vi "Calculator_Main.vi"() -> ()   [LabVIEW 2017]
uses:
  Controls/Calculator_States.ctl
  Controls/Master_Cluster.ctl
panel:
  out "Result":dbl
  out "Data Entry":string
  in  "Button 17":bool
  in  "DIV":bool
  in  "Button 21":bool
  in  "Button 20":bool
  in  "Button 19":bool
  in  "Button 18":bool
  in  "MUL":bool
  in  "SUB":bool
  in  "ADD":bool
  in  "Equals":bool
  in  "NUM 9":bool
  in  "NUM 8":bool
  in  "NUM 7":bool
  in  "NUM 6":bool
  in  "NUM 5":bool
  in  "NUM 4":bool
  in  "NUM 3":bool
  in  "NUM 2":bool
  in  "NUM 1":bool
  in  "Period":bool
  in  "NUM 0":bool
  in  "Button 1":bool
  in  "Exit":bool
  out "error out":errorcluster
  in  "error in (no error)":errorcluster
  # "CALCULATOR"
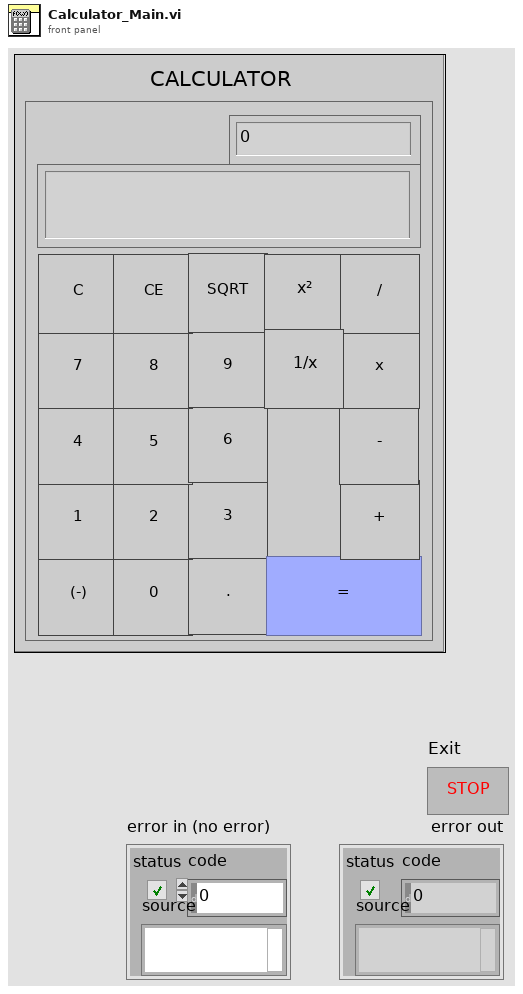
[diagram p1: front panel]
types:
  T1 = typedef "Calculator_States.ctl" = enum16{"Poll", "Initialise", "Update Data Entry", "Update Result", "Update Indicators", "Error", "Exit"}
  T2 = typedef "Master_Cluster.ctl" = cluster{"Data Entry Array":string[], "Data Entry Display":string, "Before Operator":dbl, "After Operator":dbl, "Result":dbl, "Operator":string}
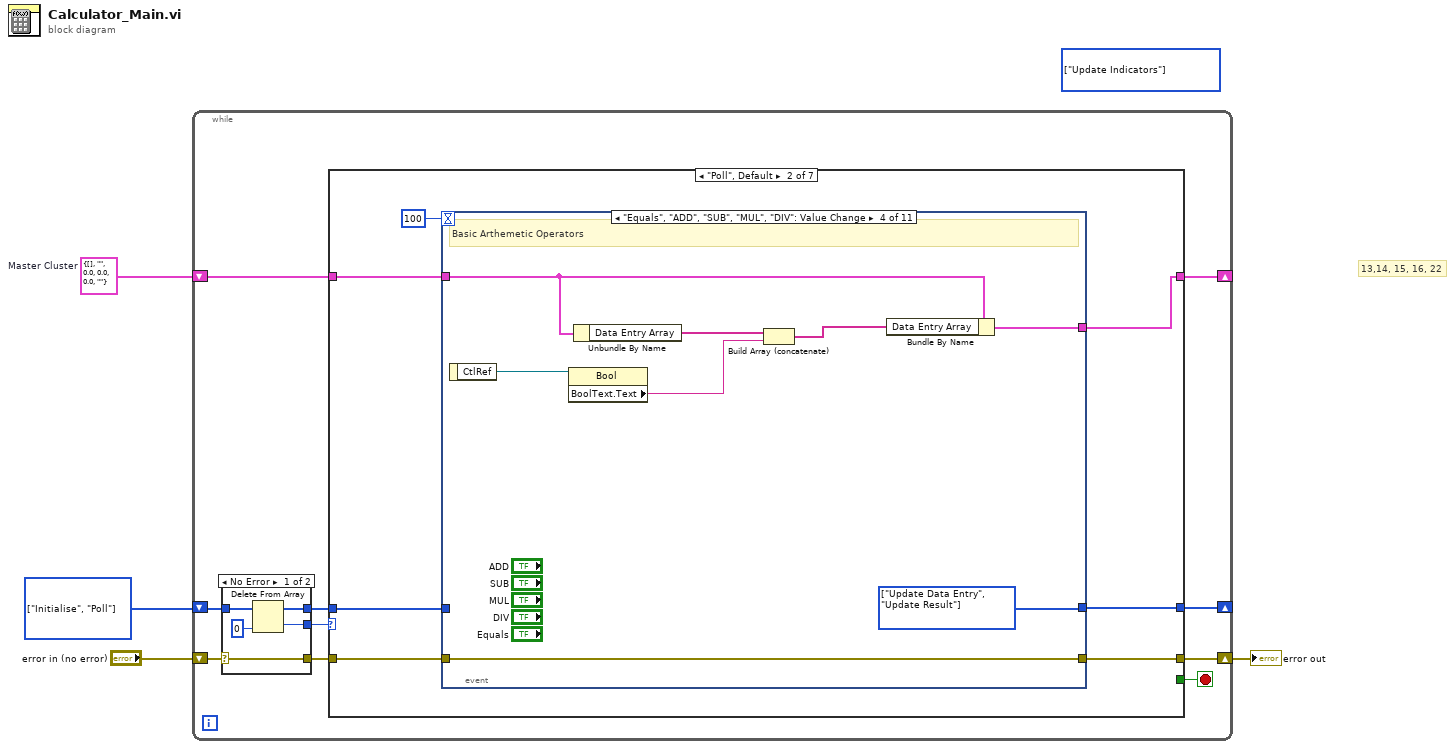
[diagram p0: block diagram]
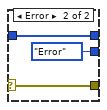
[diagram p2: hidden frame]
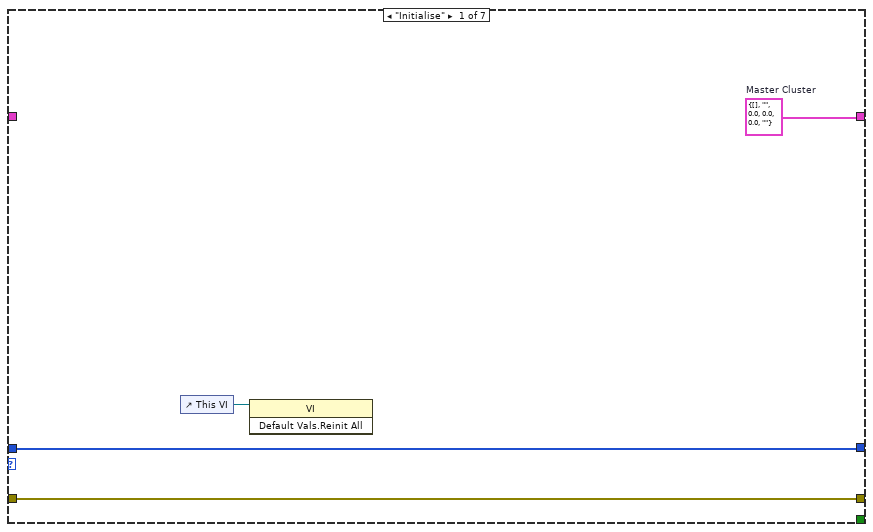
[diagram p3: hidden frame]
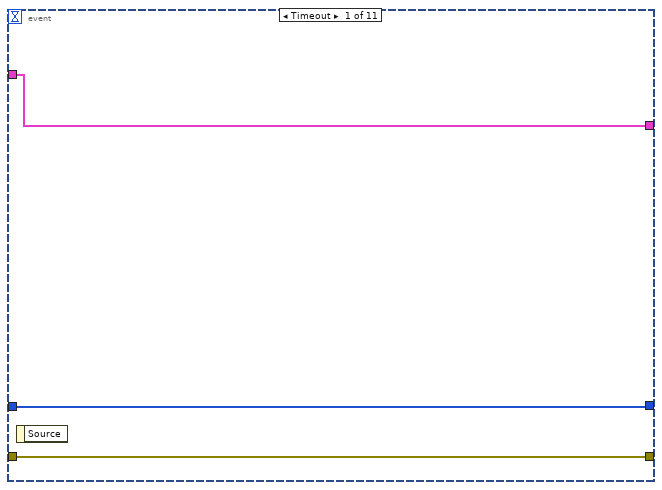
[diagram p4: hidden frame]
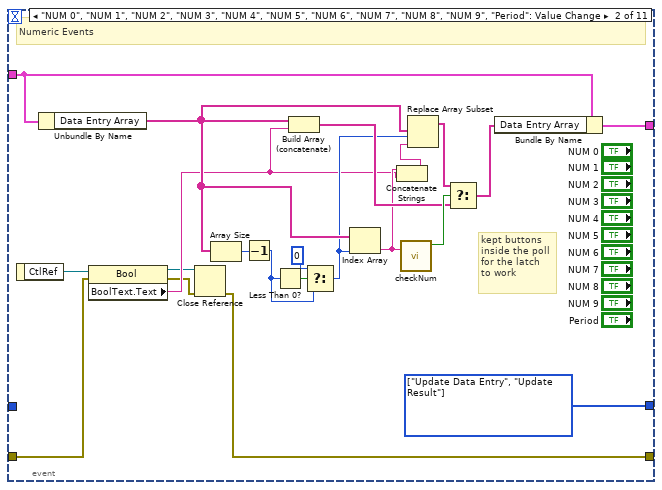
[diagram p5: hidden frame]
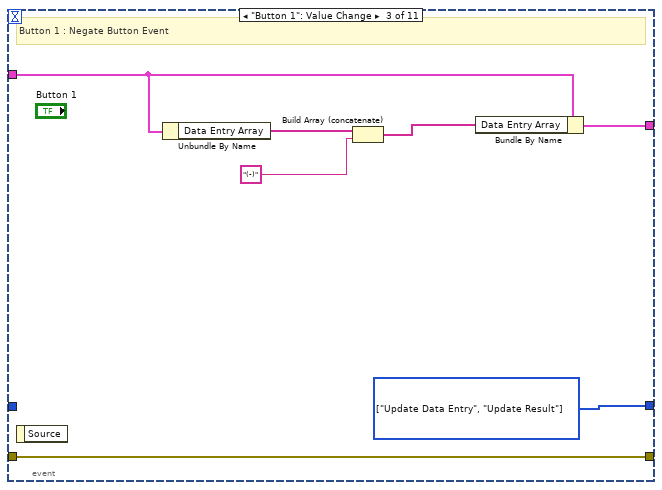
[diagram p6: hidden frame]
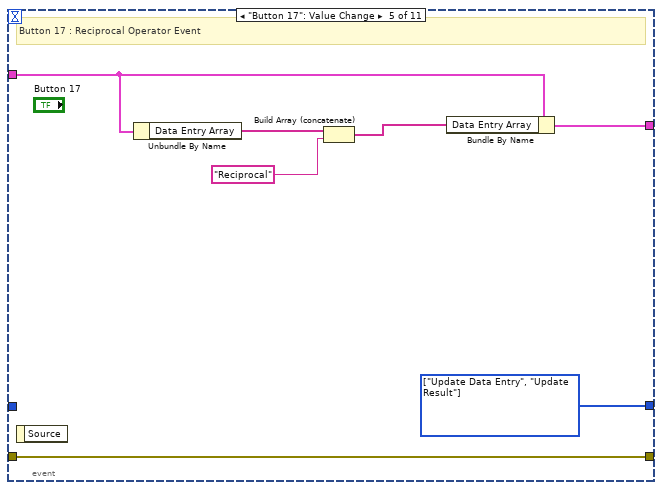
[diagram p7: hidden frame]
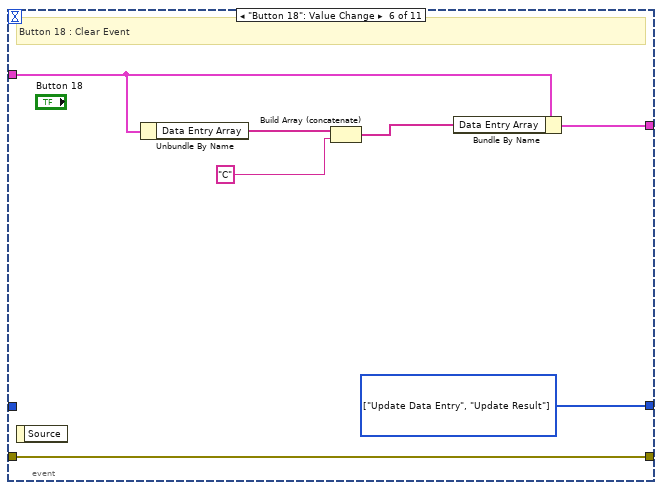
[diagram p8: hidden frame]
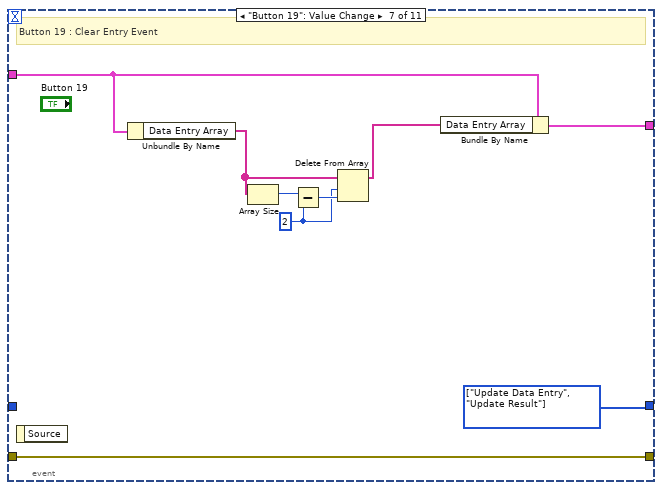
[diagram p9: hidden frame]
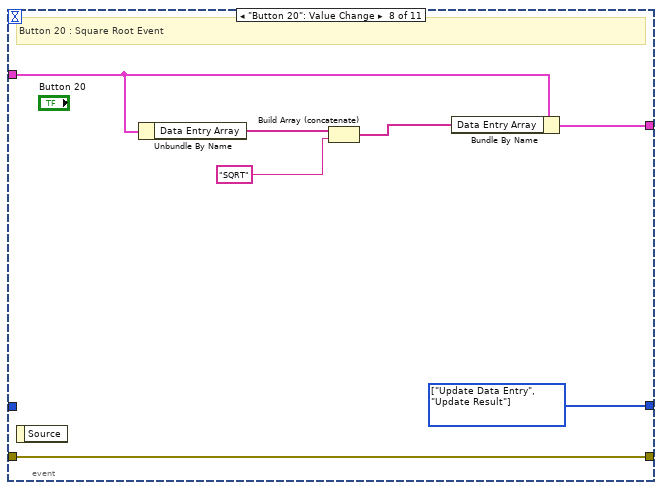
[diagram p10: hidden frame]
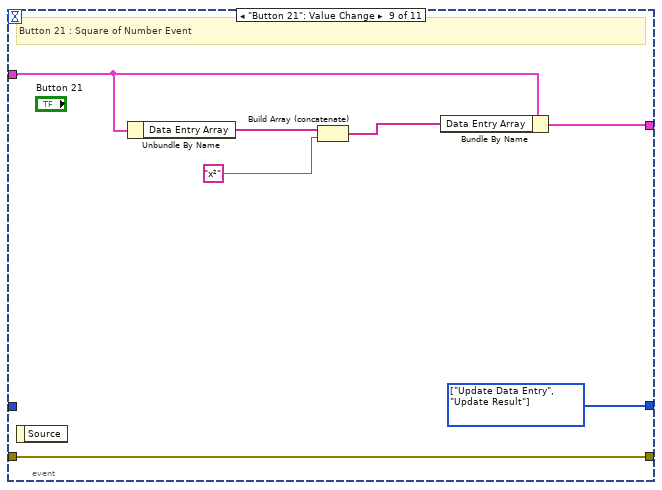
[diagram p11: hidden frame]
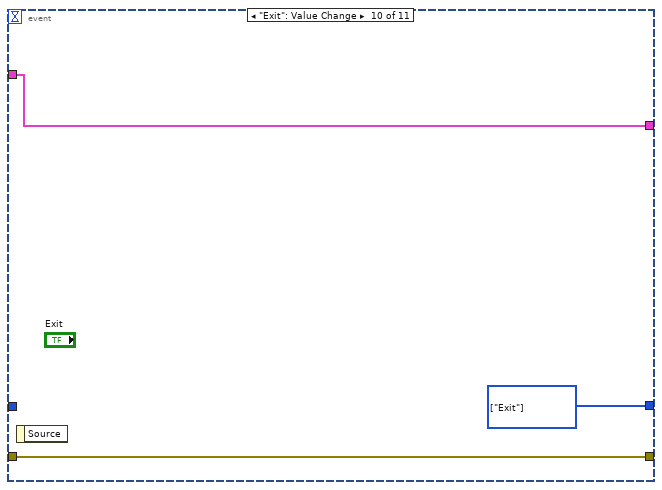
[diagram p12: hidden frame]
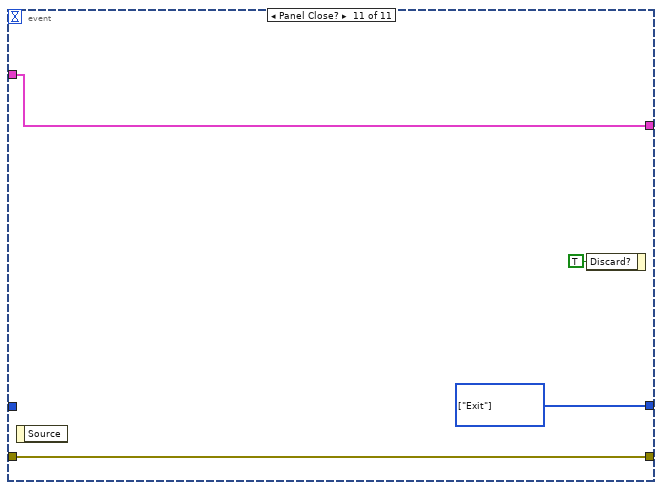
[diagram p13: hidden frame]
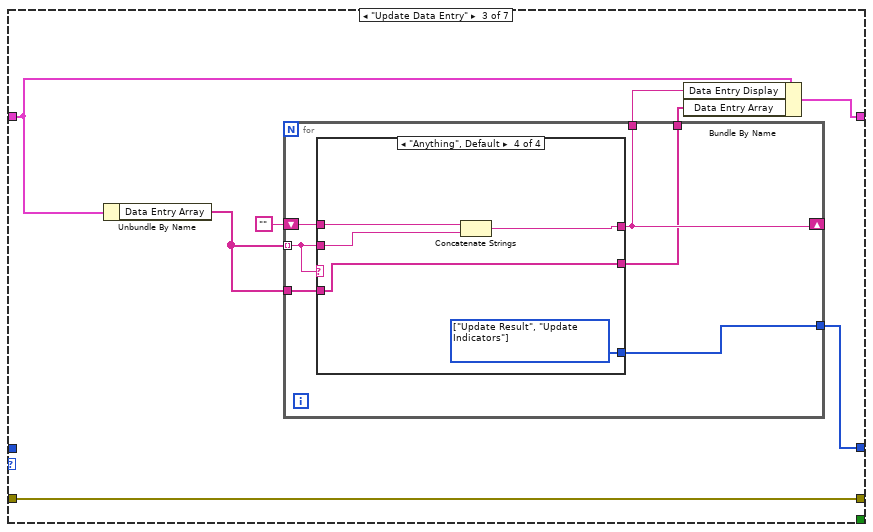
[diagram p14: hidden frame]
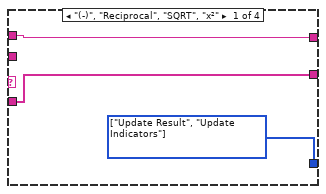
[diagram p15: hidden frame]
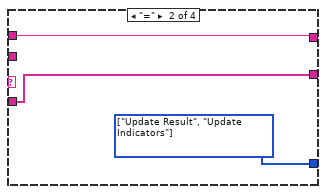
[diagram p16: hidden frame]
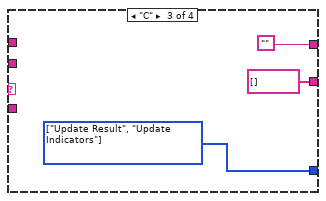
[diagram p17: hidden frame]
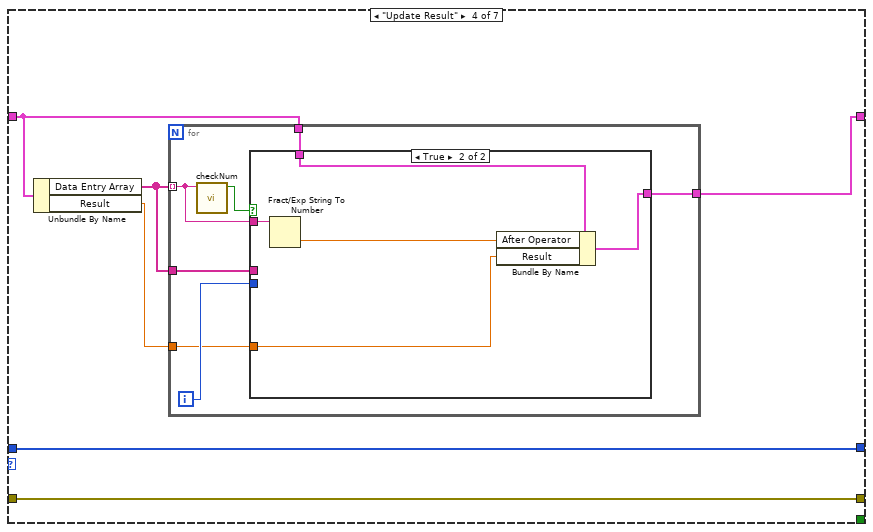
[diagram p18: hidden frame]
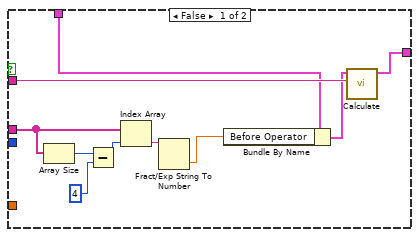
[diagram p19: hidden frame]
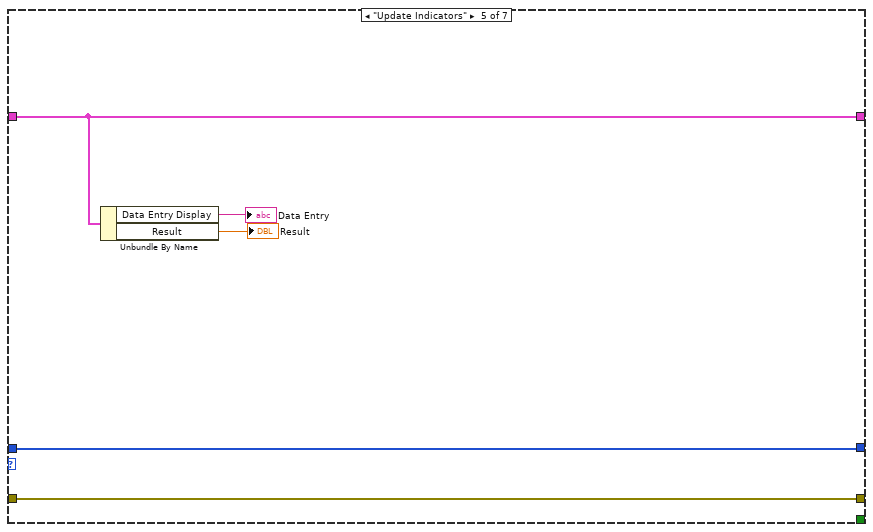
[diagram p20: hidden frame]
diagram:
  (unwired) T1[] [enum."Update Indicators"] items=["Poll", "Initialise", "Update Data Entry", "Update Result", "Update Indicators", "Error", "Exit"]
  w1 = T2 {"Data Entry Array"=[], "Data Entry Display"="", "Before Operator"=0.0, "After Operator"=0.0, "Result"=0.0, "Operator"=""}  # Master Cluster
  w4 = T1[] [enum."Initialise", enum."Poll"] items=["Poll", "Initialise", "Update Data Entry", "Update Result", "Update Indicators", "Error", "Exit"]
  # "13,14, 15, 16, 22"
  n1 = while {
    shift-right: [w10] -> w2
    shift-left: "error in (no error)" -> [w12]
    shift-right: [w7] -> _
    shift-left: w4 -> [w14]
    shift-right: [w6] -> _
    shift-left: w1 -> [w5]
    stop <- w9 stop-if-true
    n2 = case shown="No Error" w12 {
      selector: w12 -> [w18 w22]
      tunnel: [w18 w22] -> w11
      tunnel: w14 -> [w17 w20]
      tunnel: [w16 Calculator_States."Error"] -> w13
      tunnel: [w15 w20] -> w8
      frame No Error {
        n3 = Delete From Array(array=w17, index=0) -> (deleted portion=w16:T1, array with subset deleted=w15:T1[])  [unwired: 1 in]
      }
      frame Error {
      }
    }
    n4 = case shown="\"Poll\", Default" w13 {
      tunnel: w11 -> [w26 w32 w123 w150 w177 w182 w185]
      tunnel: [w26 w31 w123 w150 w177 w180 w185] -> w10
      tunnel: [_ _ _ _ _ _ TRUE] -> w9
      tunnel: w8 -> [w25 w30 _ w146 w174 w179 w184]
      tunnel: [w25 w29 w120 w146 w174 w179 w184] -> w7
      tunnel: [w23 w27 w118 w148 w176 w178 w183] -> w6
      tunnel: w5 -> [_ w28 w121 w149 w176 w178 w183]
      frame "Initialise" {
        w23 = T2 {"Data Entry Array"=[], "Data Entry Display"="", "Before Operator"=0.0, "After Operator"=0.0, "Result"=0.0, "Operator"=""}  # Master Cluster
        n5 = control-ref of="This VI"() -> (w24:refnum<vi>)
        n6 = invoke class="VI" method="Default Vals.Reinit All"(reference=w24) -> ()  [unwired: 2 in, 3 out]
      }
      frame "Poll", Default {
        n7 = event shown="[3] \"Equals\", \"ADD\", \"SUB\", \"MUL\", \"DIV\": Value Change" {
          selector: _ -> [_ _ _ _ _ _ _ _ _ _ _]
          dyn-events: _ -> [_ _ _ _ _ _ _ _ _ _ _]
          timeout: 100 -> [_ _ _ _ _ _ _ _ _ _ _]
          tunnel: w32 -> [w36 w38 w58 w68 w74 w81 w93 w97 w104 w111 w115]
          tunnel: [w36 w37 w58 w68 w74 w81 w93 w97 w104 w111 w115] -> w31
          tunnel: w30 -> [w35 _ _ _ _ _ _ _ _ _ _]
          tunnel: [w35 w55 w59 w67 w73 w80 w92 w96 w103 w112 w116] -> w29
          tunnel: w28 -> [w34 w57 w61 w70 w76 w83 w95 w99 w106 w110 w113]
          tunnel: [w34 w56 w60 w69 w75 w82 w94 w98 w105 w110 w113] -> w27
          event Timeout {
            n8 = event-data() -> ()  [unwired: 1 in, 1 out]
          }
          event "NUM 0", "NUM 1", "NUM 2", "NUM 3", "NUM 4", "NUM 5", "NUM 6", "NUM 7", "NUM 8", "NUM 9", "Period": Value Change {
            w55 = T1[] [enum."Update Data Entry", enum."Update Result"] items=["Poll", "Initialise", "Update Data Entry", "Update Result", "Update Indicators", "Error", "Exit"]
            # "kept buttons \ninside the poll\nfor the latch\nto work"
            # "Numeric Events"
            n9 = event-data() -> ("CtlRef"=w42:refnum<vi>)  [unwired: 1 in]
            n10 = Unbundle By Name(w57) -> ("Data Entry Array"=w49:string[])
            n11 = property class="Bool"(reference=w42, error in=w38) -> (reference out=w40:refnum<vi>, error out=w39:errorcluster, "BoolText.Text"=w41:string)
            n12 = Close Reference(reference=w40, error in (no error)=w39) -> (error out=w37:errorcluster)
            n13 = Array Size(array=w49) -> (size(s)=w54:i32)
            n14 = Decrement(x=w54) -> (x-1=w45:i32)
            n15 = Less Than 0?(x=w45) -> (x < 0?=w46:bool)
            n16 = Build Array (concatenate)(w49, w41) -> (w52:string[])
            n17 = Select(t=0, s=w46, f=w45) -> (s? t:f=w44:i32)
            n18 = Index Array(array=w49, index=w44) -> (element=w50:string)
            n19 = Concatenate Strings(w50, w41) -> (w47:string)
            n20 = call "checkNum.vi"("input string"=w50) -> ("Is Num"=w53:bool)  [unwired: 9 in, 1 out]
            n21 = Replace Array Subset(array=w49, new element=w47, index=w44) -> (w48:string[])
            n22 = Select(t=w48, s=w53, f=w52) -> (s? t:f=w51:string[])
            n23 = Bundle By Name(cluster=w57, "Data Entry Array"=w51) -> (w56:T2)
          }
          event "Button 1": Value Change {
            w59 = T1[] [enum."Update Data Entry", enum."Update Result"] items=["Poll", "Initialise", "Update Data Entry", "Update Result", "Update Indicators", "Error", "Exit"]
            # "Button 1 : Negate Button Event"
            n24 = event-data() -> ()  [unwired: 1 in, 1 out]
            n25 = Unbundle By Name(w61) -> ("Data Entry Array"=w64:string[])
            n26 = Build Array (concatenate)(w64, "(-)") -> (w62:string[])
            n27 = Bundle By Name(cluster=w61, "Data Entry Array"=w62) -> (w60:T2)
          }
          event "Equals", "ADD", "SUB", "MUL", "DIV": Value Change {
            w67 = T1[] [enum."Update Data Entry", enum."Update Result"] items=["Poll", "Initialise", "Update Data Entry", "Update Result", "Update Indicators", "Error", "Exit"]
            # "Basic Arthemetic Operators"
            n28 = event-data() -> ("CtlRef"=w66:refnum<vi>)  [unwired: 1 in]
            n29 = property class="Bool"(reference=w66) -> ("BoolText.Text"=w65:string)  [unwired: 1 in, 2 out]
            n30 = Unbundle By Name(w70) -> ("Data Entry Array"=w72:string[])
            n31 = Build Array (concatenate)(w72, w65) -> (w71:string[])
            n32 = Bundle By Name(cluster=w70, "Data Entry Array"=w71) -> (w69:T2)
          }
          event "Button 17": Value Change {
            w73 = T1[] [enum."Update Data Entry", enum."Update Result"] items=["Poll", "Initialise", "Update Data Entry", "Update Result", "Update Indicators", "Error", "Exit"]
            # "Button 17 : Reciprocal Operator Event"
            n33 = event-data() -> ()  [unwired: 1 in, 1 out]
            n34 = Unbundle By Name(w76) -> ("Data Entry Array"=w79:string[])
            n35 = Build Array (concatenate)(w79, "Reciprocal") -> (w77:string[])
            n36 = Bundle By Name(cluster=w76, "Data Entry Array"=w77) -> (w75:T2)
          }
          event "Button 18": Value Change {
            w80 = T1[] [enum."Update Data Entry", enum."Update Result"] items=["Poll", "Initialise", "Update Data Entry", "Update Result", "Update Indicators", "Error", "Exit"]
            # "Button 18 : Clear Event"
            n37 = event-data() -> ()  [unwired: 1 in, 1 out]
            n38 = Unbundle By Name(w83) -> ("Data Entry Array"=w86:string[])
            n39 = Build Array (concatenate)(w86, "C") -> (w84:string[])
            n40 = Bundle By Name(cluster=w83, "Data Entry Array"=w84) -> (w82:T2)
          }
          event "Button 19": Value Change {
            w89 = 2 ("y")
            w92 = T1[] [enum."Update Data Entry", enum."Update Result"] items=["Poll", "Initialise", "Update Data Entry", "Update Result", "Update Indicators", "Error", "Exit"]
            # "Button 19 : Clear Entry Event"
            n41 = event-data() -> ()  [unwired: 1 in, 1 out]
            n42 = Unbundle By Name(w95) -> ("Data Entry Array"=w87:string[])
            n43 = Array Size(array=w87) -> (size(s)=w91:i32)
            n44 = Subtract(x=w91, y=w89) -> (x-y=w90:i32)
            n45 = Delete From Array(array=w87, length=w89, index=w90) -> (array with subset deleted=w88:string[])  [unwired: 1 out]
            n46 = Bundle By Name(cluster=w95, "Data Entry Array"=w88) -> (w94:T2)
          }
          event "Button 20": Value Change {
            w96 = T1[] [enum."Update Data Entry", enum."Update Result"] items=["Poll", "Initialise", "Update Data Entry", "Update Result", "Update Indicators", "Error", "Exit"]
            # "Button 20 : Square Root Event"
            n47 = event-data() -> ()  [unwired: 1 in, 1 out]
            n48 = Unbundle By Name(w99) -> ("Data Entry Array"=w102:string[])
            n49 = Build Array (concatenate)(w102, "SQRT") -> (w100:string[])
            n50 = Bundle By Name(cluster=w99, "Data Entry Array"=w100) -> (w98:T2)
          }
          event "Button 21": Value Change {
            w103 = T1[] [enum."Update Data Entry", enum."Update Result"] items=["Poll", "Initialise", "Update Data Entry", "Update Result", "Update Indicators", "Error", "Exit"]
            # "Button 21 : Square of Number Event"
            n51 = event-data() -> ()  [unwired: 1 in, 1 out]
            n52 = Unbundle By Name(w106) -> ("Data Entry Array"=w109:string[])
            n53 = Build Array (concatenate)(w109, "x²") -> (w107:string[])
            n54 = Bundle By Name(cluster=w106, "Data Entry Array"=w107) -> (w105:T2)
          }
          event "Exit": Value Change {
            w112 = T1[] [enum."Exit"] items=["Poll", "Initialise", "Update Data Entry", "Update Result", "Update Indicators", "Error", "Exit"]
            n55 = event-data() -> ()  [unwired: 1 in, 1 out]
          }
          event Panel Close? {
            w116 = T1[] [enum."Exit"] items=["Poll", "Initialise", "Update Data Entry", "Update Result", "Update Indicators", "Error", "Exit"]
            n56 = event-data() -> ()  [unwired: 1 in, 1 out]
            n57 = event-data("Discard?"=TRUE) -> ()  [unwired: 1 in, 1 out]
          }
        }
      }
      frame "Update Data Entry" {
        n58 = Unbundle By Name(w121) -> ("Data Entry Array"=w122:string[])
        n59 = for {
          shift-right: [w126] -> _
          shift-left: "" -> [w130]
          tunnel: w122 -> [w129] mode=indexing
          tunnel: w122 -> [w128]
          tunnel: [w127] -> w120
          tunnel: [w126] -> w119
          tunnel: [w125] -> w117
          n60 = case shown="\"Anything\", Default" w129 {
            tunnel: w130 -> [w133 w135 _ w144]
            tunnel: w129 -> [_ _ _ w142]
            tunnel: [w133 w135 "" w143] -> w126
            tunnel: w128 -> [w131 w134 _ w140]
            tunnel: [w132 w136 w138 w141] -> w127
            tunnel: [w131 w134 string[] [] ("Data Entry Array") w140] -> w125
            frame "(-)", "Reciprocal", "SQRT", "x²" {
              w132 = T1[] [enum."Update Result", enum."Update Indicators"] items=["Poll", "Initialise", "Update Data Entry", "Update Result", "Update Indicators", "Error", "Exit"]
            }
            frame "=" {
              w136 = T1[] [enum."Update Result", enum."Update Indicators"] items=["Poll", "Initialise", "Update Data Entry", "Update Result", "Update Indicators", "Error", "Exit"]
            }
            frame "C" {
              w138 = T1[] [enum."Update Result", enum."Update Indicators"] items=["Poll", "Initialise", "Update Data Entry", "Update Result", "Update Indicators", "Error", "Exit"]
            }
            frame "Anything", Default {
              w141 = T1[] [enum."Update Result", enum."Update Indicators"] items=["Poll", "Initialise", "Update Data Entry", "Update Result", "Update Indicators", "Error", "Exit"]
              n61 = Concatenate Strings(w144, w142) -> (w143:string)
            }
          }
        }
        n62 = Bundle By Name(cluster=w121, "Data Entry Display"=w119, "Data Entry Array"=w117) -> (w118:T2)
      }
      frame "Update Result" {
        n63 = Unbundle By Name(w149) -> ("Data Entry Array"=w147:string[], "Result"=w145:dbl)
        n64 = for {
          tunnel: w147 -> [w154] mode=indexing
          tunnel: w149 -> [w156]
          tunnel: [w155] -> w148
          tunnel: w147 -> [w152]
          tunnel: w145 -> [w151]
          i -> [w153]
          n65 = call "checkNum.vi"("input string"=w154) -> ("Is Num"=w157:bool)  [unwired: 9 in, 1 out]
          n66 = case shown="True" w157 {
            tunnel: w156 -> [w164 w170]
            tunnel: [w166 w169] -> w155
            tunnel: w154 -> [w167 w171]
            tunnel: w152 -> [w165 _]
            tunnel: w153 -> [_ _]
            tunnel: w151 -> [_ w168]
            frame False {
              n67 = Array Size(array=w165) -> (size(s)=w159:i32)
              n68 = Subtract(x=w159, y=4) -> (x-y=w160:i32)
              n69 = Index Array(array=w165, index=w160) -> (element=w162:string)
              n70 = Fract/Exp String To Number(string=w162) -> (number=w161:dbl)  [unwired: 3 in, 1 out]
              n71 = Bundle By Name(cluster=w164, "Before Operator"=w161) -> (w163:T2)
              n72 = call "Calculate.vi"("Input String"=w167, "Master Cluster"=w163) -> ("Output M Cluster"=w166:T2)  [unwired: 6 in, 3 out]
            }
            frame True {
              n73 = Fract/Exp String To Number(string=w171) -> (number=w172:dbl)  [unwired: 3 in, 1 out]
              n74 = Bundle By Name(cluster=w170, "After Operator"=w172, "Result"=w168) -> (w169:T2)
            }
          }
        }
      }
      frame "Update Indicators" {
        n75 = Unbundle By Name(w176) -> ("Data Entry Display"=→"Data Entry":string, "Result"=→"Result":dbl)
      }
      frame "Error" {
        n76 = call <vilib>:"Simple Error Handler.vi"("error in (no error)"=w182) -> ("error out"=w181:errorcluster)  [unwired: 4 in, 4 out]
        n77 = call <vilib>:"Clear Errors.vi"("error in (no error)"=w181) -> ("error out"=w180:errorcluster)  [unwired: 5 in, 1 out]
      }
      frame "Exit" {
      }
    }
  }
  "error out" <- w2
